vi "GetType.vi"(8 "error in (no error)":errorcluster, 11 "Read All Sensor Data Msg":refnum<class "Read All Sensor Data Msg.lvclass">) -> (0 "error out":errorcluster, 2 "Data Sample":variant, 3 "Read All Sensor Data Msg":refnum<class "Read All Sensor Data Msg.lvclass">)   [LabVIEW 2016, in "LS218.lvlib" / "Read All Sensor Data Msg.lvclass"]
uses:
  Read All Sensor Data Msg.lvclass
  Read All Sensor Data Msg.lvclass/Read All Sensor Data Msg.ctl
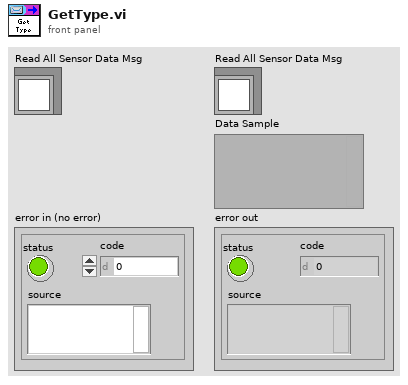
[diagram p1: front panel]
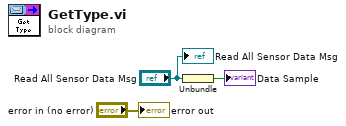
[diagram p0: block diagram]
diagram:
  n1 = Unbundle("Read All Sensor Data Msg") -> (→"Data Sample":bool)
  "error out" <- "error in (no error)"
  "Read All Sensor Data Msg" <- "Read All Sensor Data Msg"
